vi "D2SParser - Private - Function - Read Character Level.vi"(8 "error in (no error)":errorcluster, 11 "D2SParser in":refnum<class "D2SParser.lvclass">) -> (0 "error out":errorcluster, 3 "D2SParser out":refnum<class "D2SParser.lvclass">)   [LabVIEW 2015, in "D2SParser.lvclass"]
uses:
  D2SParser.lvclass
  D2SParser.lvclass/D2SParser.ctl
  D2Character/D2Character.lvclass/D2Character.ctl
  D2Character/D2Character - Accessors - Set Level.vi
  D2SParser - Private - Helper - Read Byte.vi
  D2Character/D2Character.lvclass
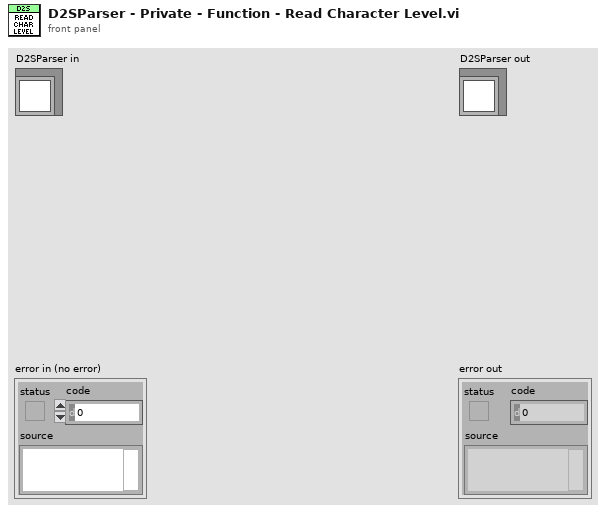
[diagram p1: front panel]
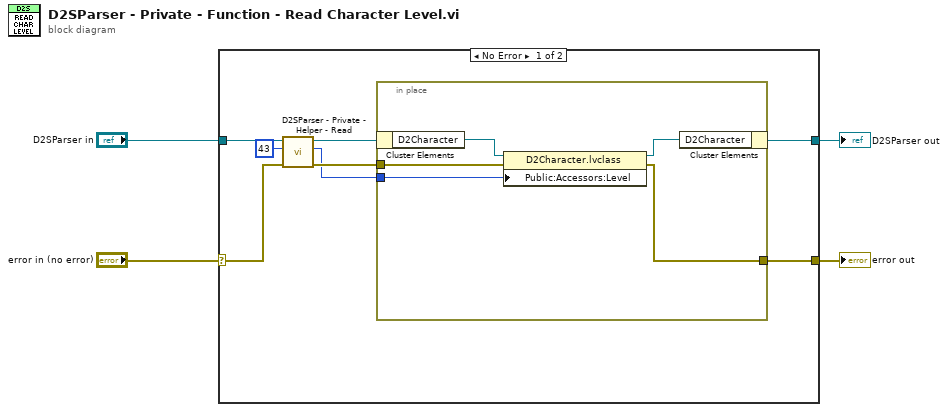
[diagram p0: block diagram]
diagram:
  n1 = case shown="No Error" "error in (no error)" {
    selector: "error in (no error)" -> [w11 w19]
    tunnel: [w8 w19] -> w3
    tunnel: [w7 w18] -> w1
    tunnel: "D2SParser in" -> [w12 w18]
    frame No Error {
      n2 = call-poly "D2SParser - Private - Helper - Read.vi"("error in (no error)"=w11, "Position"=i64 43, "D2SParser in"=w12) -> ("error out"=w9:errorcluster, "byte"=w5:u8, "D2SParser out"=w10:refnum<class "D2SParser.lvclass">)  [unwired: 6 in]
      n3 = in-place {
        in-place-border: w9 -> [w15]
        in-place-border: [w14] -> w8
        in-place-border: w5 -> [w13]
        n4 = in-place-cluster #1(w10) -> ("D2Character"=w17:refnum<class "D2Character.lvclass">)
        n5 = property class="D2Character.lvclass"(reference=w17, error in=w15, "Public:Accessors:Level"=w13) -> (reference out=w16:refnum<class "D2Character.lvclass">, error out=w14:errorcluster)
        n6 = in-place-cluster #1("D2Character"=w16) -> (w7:refnum<class "D2SParser.lvclass">)
      }
    }
    frame Error {
    }
  }
  "error out" <- w3
  "D2SParser out" <- w1
